vi "AWS Process Command.vi"(8 "error in":errorcluster, 11 "LV-Data.AWS CLI":refnum<class "LV-Data.AWS CLI.lvclass">) -> (0 "error out":errorcluster, 2 "command line":string, 3 "LV-Data.AWS CLI out":refnum<class "LV-Data.AWS CLI.lvclass">)   [LabVIEW 2019, in "LV-Data.AWS CLI.lvclass"]
uses:
  LV-Data.AWS CLI.lvclass
  LV-Data.AWS CLI.lvclass/LV-Data.AWS CLI.ctl
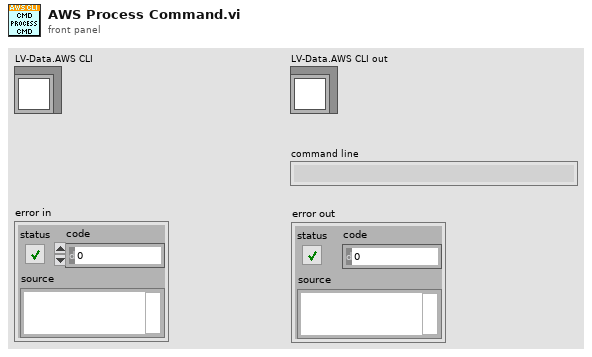
[diagram p1: front panel]
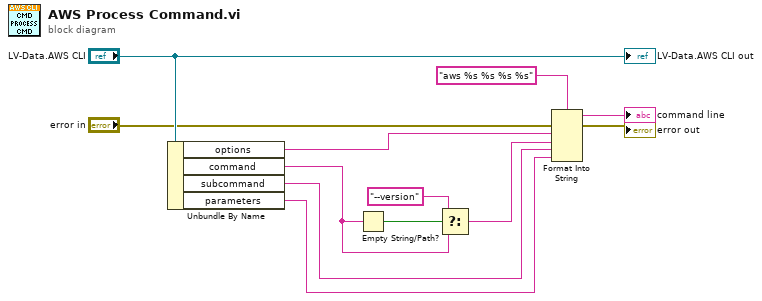
[diagram p0: block diagram]
diagram:
  n1 = Unbundle By Name("LV-Data.AWS CLI") -> ("options"=w7:string, "command"=w6:string, "subcommand"=w5:string, "parameters"=w4:string)
  n2 = Empty String/Path?(string/path=w6) -> (empty?=w10:bool)
  n3 = Select(t="--version", s=w10, f=w6) -> (s? t:f=w8:string)
  n4 = Format Into String(format string="aws %s %s %s %s", error in="error in", w7, w8, w5, w4) -> (resulting string=→"command line":string, error out=→"error out":errorcluster)  [unwired: 1 in]
  "LV-Data.AWS CLI out" <- "LV-Data.AWS CLI"
